vi "tarea.vi"() -> ()   [LabVIEW 2016]
panel:
  out "W":bool
  out "X":bool
  out "Y":bool
  out "Z":bool
  in  "A":bool
  in  "B":bool
  in  "C":bool
  in  "D":bool
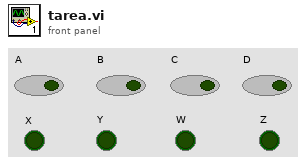
[diagram p1: front panel]
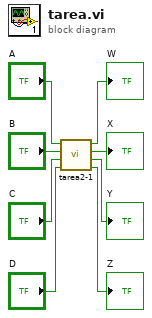
[diagram p0: block diagram]
diagram:
  n1 = call <userlib>:"tarea2-1.vi"("D"="D", "C"="C", "B"="B", "A"="A") -> ("Z"=→"Z":bool, "Y"=→"Y":bool, "X"=→"X":bool, "W"=→"W":bool)
